vi "play-analyze-z-axis.vi"() -> ()   [LabVIEW 2015]
uses:
  <vilib>/userdefined/High Color/nirio_resource_hc.ctl
  <vilib>/FPGAPlugInAG/cRIO-9082/niLvFpga_Open_cRIO-9082.vi
  <vilib>/rvi/interface/common/dynamic/niFpgaDynamicAddResources.vi
  <vilib>/FPGAPlugInAG/Dynamic/niLvFpga_Reset_Dynamic.vi
  <vilib>/rvi/interface/common/niFpgaWaitOnOcc.vi
  <vilib>/Utility/error.llb/Error Cluster From Error Code.vi
  <vilib>/rvi/errors/niLvFpgaAdjustHostInterfaceError.vi
  <vilib>/FPGAPlugInAG/Dynamic/niLvFpga_Run_Dynamic.vi
  <vilib>/Utility/file.llb/Write To Spreadsheet File (DBL).vi
  <vilib>/FPGAPlugInAG/Dynamic/niLvFpga_Close_Dynamic.vi
  <vilib>/rvi/interface/nirviOpenFPGA/nirviOpenFPGA.xnode
  FPGA Bitfiles/afmimagingcontro_FPGATargetSPARTA_analyze-z-axis_yYroOCuDKm4.lvbitx
  <vilib>/rvi/interface/nirviMethod/nirviMethod.xnode
  <vilib>/rvi/interface/nirviReadWriteControl/nirviReadWriteControl.xnode
  <vilib>/rvi/interface/nirviCloseFPGA/nirviCloseFPGA.xnode
  <vilib>/rvi/errors/niLvFpgaMergeErrorWithErrorCode.vi
  <vilib>/FPGAPlugInAG/Dynamic/niLvFpga_ReadFifo_Dynamic.vi
  NiFpgaLv.dll
  <vilib>/rvi/interface/Simulation/niFpgaSimulationCallBeginRW.vi
  <vilib>/FPGAPlugInAG/Dynamic/niLvFpga_ConfigureFifo_Dynamic.vi
panel:
  in  "ABORT":bool
  out "Numeric":i32
  out "currentCase":i16
  out "caseiter":i16
  in  "trigger-0":bool
  out "Mod2/AI2":fxp<+/-,24,5>
  out "u(k)":sgl
  in  "init Z up":sgl
  in  "ramp-rate":sgl=-5e-06
  in  "initial-case":u8
  in  "Ki":sgl=0.001
  in  "setpoint":sgl
  in  "nsamps":i32
  out "Waveform Graph":dbl[](graph)
  in  "outputData BOTH":path=path "C:/Users/arnold/Documents/labview/afm_imaging/data/analyze-z-axis-PIon.csv"
  out "y iter":i32
  out "size(s)":i32
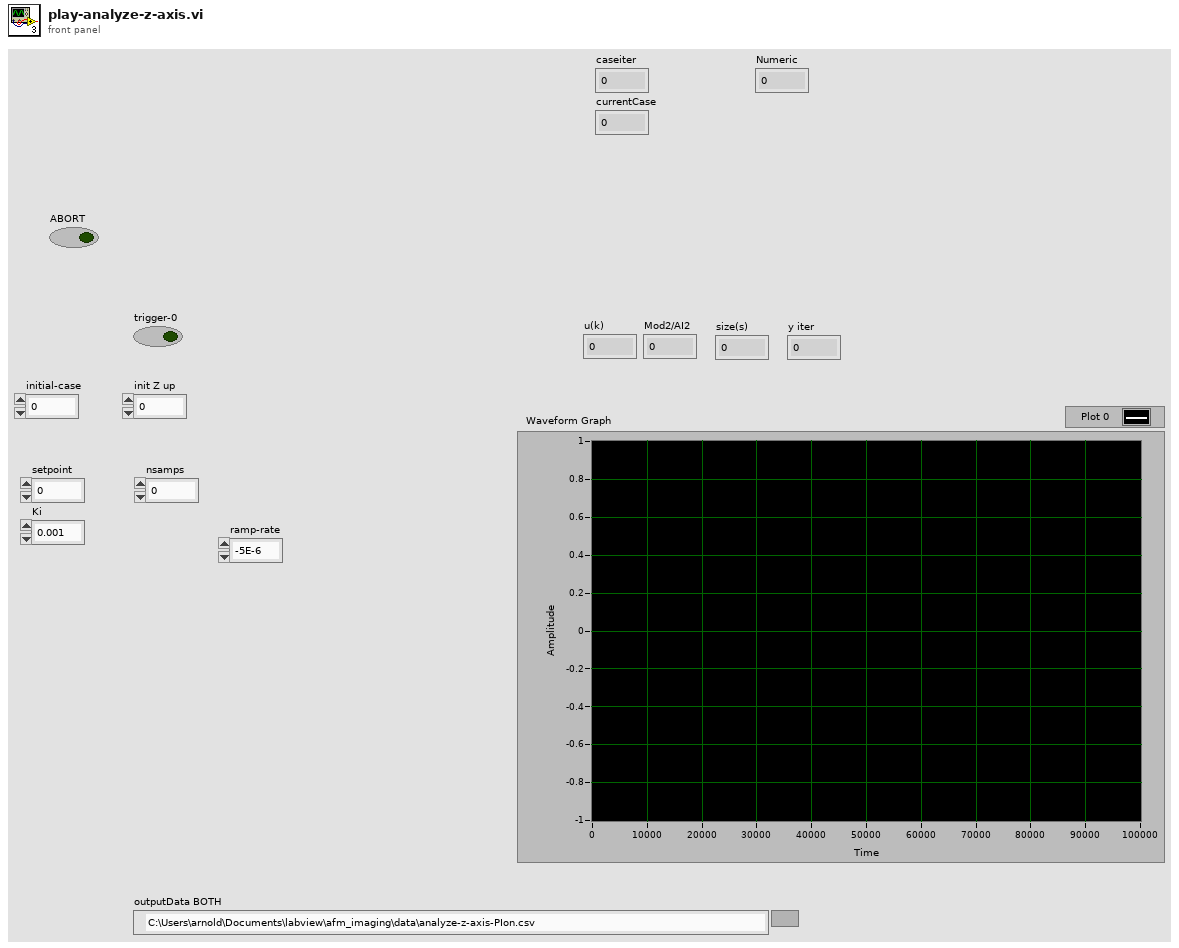
[diagram p1: front panel]
types:
  T1 = typedef "nirio_resource_hc.ctl" = tag
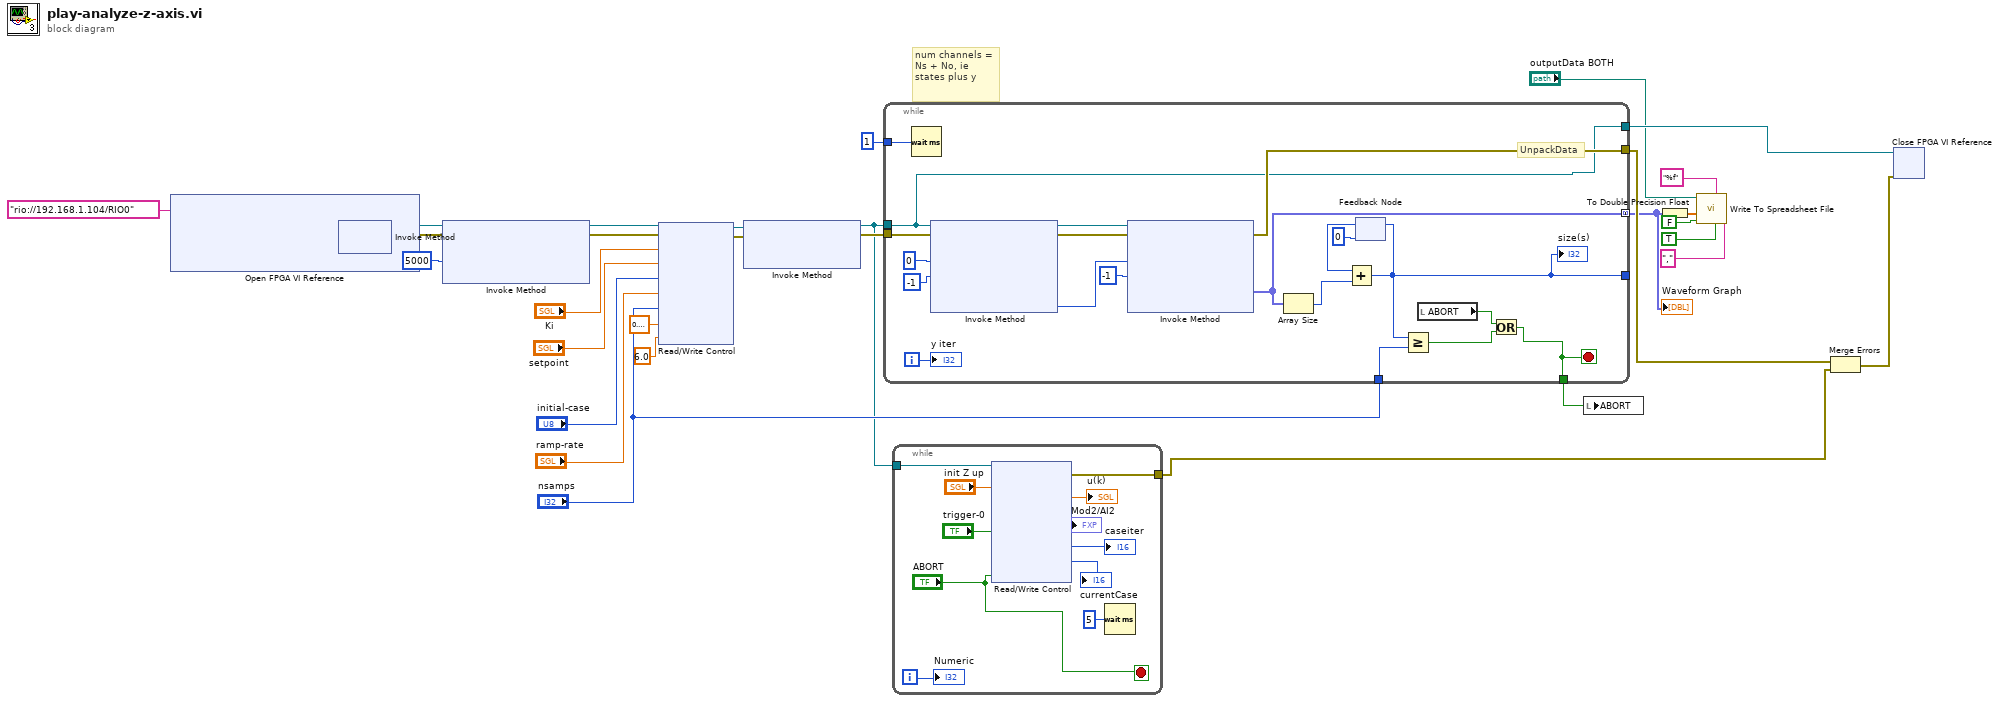
[diagram p0: block diagram]
diagram:
  # "num channels = Ns + No, ie states plus y"
  n1 = xnode "Open FPGA VI Reference"("resource name"=T1 "rio://192.168.1.104/RIO0") -> ("FPGA VI Reference Out"=w29:refnum<k20>, "error out"=w28:errorcluster)  [unwired: 1 in]
  n2 = xnode "Invoke Method"("FPGA VI Reference In"=w29, "error in"=w28) -> ("FPGA VI Reference Out"=w20:refnum<k20>, "error out"=w19:errorcluster)
  n3 = xnode "Invoke Method"("FPGA VI Reference In"=w20, "error in"=w19, "Requested Depth"=5000) -> ("FPGA VI Reference Out"=w18:refnum<k20>, "error out"=w17:errorcluster)  [unwired: 1 out]
  n4 = xnode "Read/Write Control"("FPGA VI Reference In"=w18, "error in"=w17, "Ki"="Ki", "setpoint"="setpoint", "initial-case"="initial-case", "ramp-rate"="ramp-rate", "numIters"="nsamps", "TOL"=sgl 0.3, "uz-max"=sgl 6.0) -> ("FPGA VI Reference Out"=w15:refnum<k20>, "error out"=w16:errorcluster)
  n5 = xnode "Invoke Method"("FPGA VI Reference In"=w15, "error in"=w16) -> ("FPGA VI Reference Out"=w9:refnum<k20>, "error out"=w21:errorcluster)  [unwired: 1 in]
  n6 = while {
    tunnel: 1 -> [w52]
    tunnel: w9 -> [w36]
    tunnel: w21 -> [w39]
    tunnel: [w45] -> w5
    tunnel: [w36] -> w31
    tunnel: [w42] -> w1 mode=concatenating
    tunnel: [w37] -> _
    tunnel: "nsamps" -> [w38]
    tunnel: [w33] -> w3
    i -> [w44]
    stop <- w33 stop-if-true
    # "UnpackData"
    n7 = Wait (ms)(milliseconds to wait=w52) -> ()  [unwired: 1 out]
    n8 = xnode "Invoke Method"("FPGA VI Reference In"=w36, "error in"=w39, "Number of Elements"=0 ("Timeout (ms)"), "Timeout (ms)"=-1) -> ("FPGA VI Reference Out"=w48:refnum<k20>, "error out"=w49:errorcluster, "Elements Remaining"=w43:u32)  [unwired: 1 out]
    n9 = xnode "Invoke Method"("FPGA VI Reference In"=w48, "error in"=w49, "Number of Elements"=w43, "Timeout (ms)"=-1) -> ("error out"=w45:errorcluster, "Data"=w42:fxp<+/-,16,5>[])  [unwired: 2 out]
    n10 = Array Size(array=w42) -> (size(s)=w41:i32)
    n11 = feedback #1(0) -> (w40:i32)
    n12 = Add(x=w40, y=w41) -> (x+y=w37:i32)
    "size(s)" <- w37
    n13 = feedback-in #1(w37) -> ()
    n14 = Greater Or Equal?(x=w37, y=w38) -> (x >= y?=w34:bool)
    n15 = local read "ABORT"() -> (w35:bool)
    n16 = Or(x=w35, y=w34) -> (x .or. y?=w33:bool)
    "y iter" <- w44
  }
  "Waveform Graph" <- w1
  n17 = while {
    tunnel: w9 -> [w63]
    tunnel: [w59] -> w6
    i -> [w54]
    stop <- "ABORT" stop-if-true
    n18 = xnode "Read/Write Control"("FPGA VI Reference In"=w63, "init Z up"="init Z up", "trigger-0"="trigger-0", "stop"="ABORT") -> ("error out"=w59:errorcluster, "u(k)"=→"u(k)":sgl, "Mod2/AI2"=→"Mod2/AI2":fxp<+/-,24,5>, "caseiter"=→"caseiter":i16, "currentCase"=→"currentCase":i16)  [unwired: 1 in, 1 out]
    n19 = Wait (ms)(milliseconds to wait=u32 5) -> ()  [unwired: 1 out]
    "Numeric" <- w54
  }
  n20 = local write "ABORT"(w3) -> ()
  n21 = To Double Precision Float(number=w1) -> (double precision float=w2:dbl[])
  n22 = call-poly <vilib>:"Write To Spreadsheet File.vi"("delimiter (\\t)"=",", "transpose? (no:F)"=TRUE, "format (%.3f)"="%f", "append to file? (new file:F)"=FALSE, "1D data"=w2, "file path (dialog if empty)"="outputData BOTH") -> ()  [unwired: 2 in, 1 out]
  n23 = Merge Errors(w5, w6) -> (w4:errorcluster)
  n24 = xnode "Close FPGA VI Reference"("FPGA VI Reference In"=w31, "error in"=w4) -> ()  [unwired: 1 out]
